vi "ADS Launcher.vi"(8 "error in (no error)":errorcluster) -> (0 "error out":errorcluster)   [LabVIEW 2018, in "ADS Actor.lvlib" / "ADS.lvclass"]
uses:
  ADS.lvclass
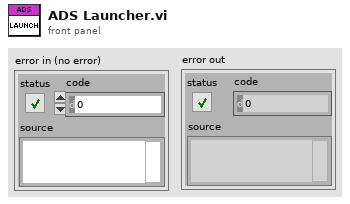
[diagram p1: front panel]
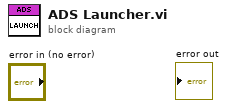
[diagram p0: block diagram]
diagram:
